vi "Read Roles.vi"(8 "error in (no error)":errorcluster, 11 "NormalDefensivePlay in":refnum<class "NormalDefensivePlay.lvclass">) -> (0 "error out":errorcluster, 2 "Roles":T1, 3 "NormalDefensivePlay out":refnum<class "NormalDefensivePlay.lvclass">)   [LabVIEW 2023, in "NormalDefensivePlay.lvclass"]
uses:
  NormalDefensivePlay.lvclass
  DefenderAreaRole_class/DefenderAreaRole.lvclass
  NormalDefensivePlay.lvclass/NormalDefensivePlay.ctl
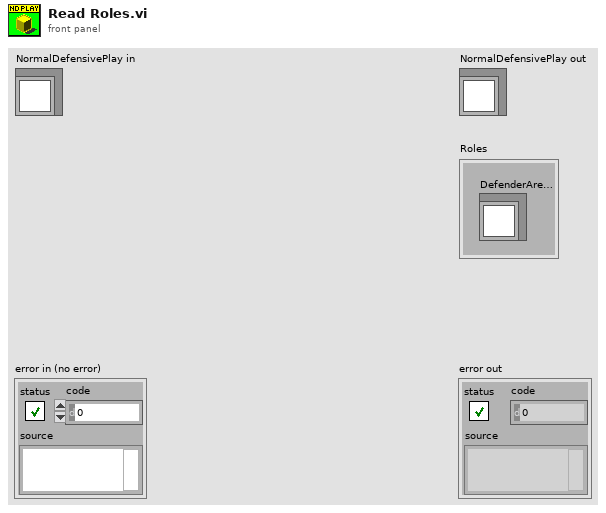
[diagram p1: front panel]
types:
  T1 = cluster{"DefenderAreaRole":refnum<class "DefenderAreaRole.lvclass">}
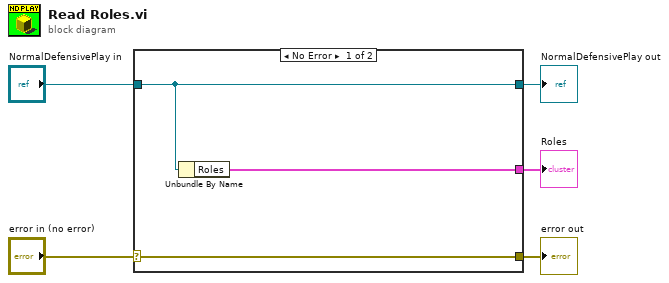
[diagram p0: block diagram]
diagram:
  n1 = case shown="No Error" "error in (no error)" {
    selector: "error in (no error)" -> [w8 w9]
    tunnel: [w8 w9] -> w4
    tunnel: [w7 w10] -> w2
    tunnel: "NormalDefensivePlay in" -> [w7 w10]
    tunnel: [w6 _] -> w1
    frame No Error {
      n2 = Unbundle By Name(w7) -> ("Roles"=w6:T1)
    }
    frame Error {
    }
  }
  "error out" <- w4
  "NormalDefensivePlay out" <- w2
  "Roles" <- w1
